vi "INIT.vi"(8 "error in (no error)":errorcluster, 11 "DAQmxTaskContainer in":refnum<class "DAQmxTaskContainer.lvclass">) -> (0 "error out":errorcluster, 3 "DAQmxTaskContainer out":refnum<class "DAQmxTaskContainer.lvclass">)   [LabVIEW 2015, in "DAQmxTaskContainer.lvclass"]
uses:
  DAQmxTaskContainer.lvclass
  dependecies/ControlsVIs/Clusters-def/SERVER-Commands.ctl
  dependecies/ControlsVIs/Clusters-def/Message types.ctl
  DAQmxTaskContainer_General/DAQmxTaksContainer_General.lvclass/DAQmxTaksContainer_General.ctl
  DAQmxTask.lvclass/DAQmxTask.ctl
  DAQmxTaskContainer_General/DAQmxTaksContainer_General.lvclass
  DAQmxTask.lvclass
  Control/Control-Server/Control-Server.lvclass
  Message/Message.lvclass
  GeneralFunctionality/GeneralFunctionality.lvclass
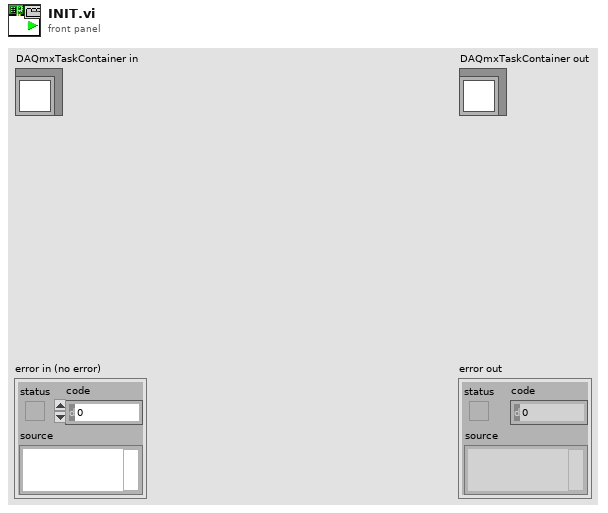
[diagram p1: front panel]
types:
  T1 = typedef "Message types.ctl" = string
  T2 = typedef "Control-Server.lvclass/SERVER-Commands.ctl" = string
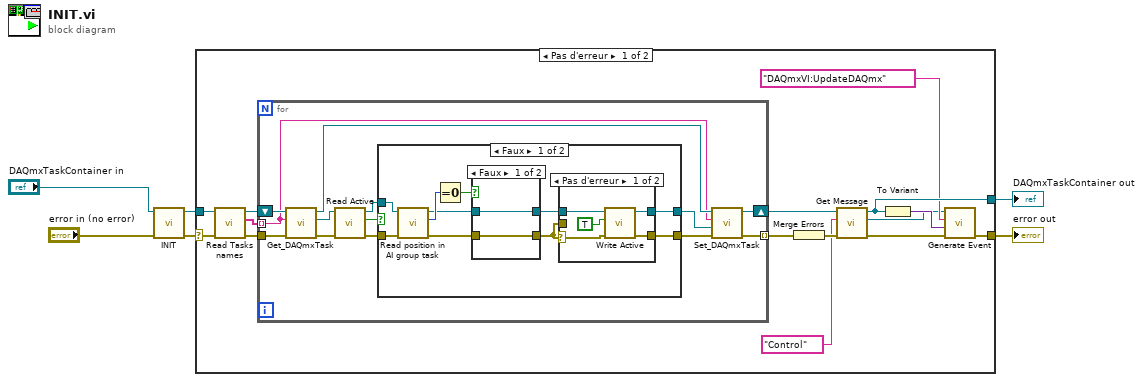
[diagram p0: block diagram]
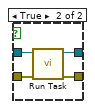
[diagram p2: hidden frame]
diagram:
  n1 = call-parent "INIT.vi"("error in (no error)"="error in (no error)", "DAQmxTaksContainer_General in"="DAQmxTaskContainer in") -> ("error out"=w4:errorcluster, "DAQmxTaksContainer_General out"=w2:refnum<class "DAQmxTaskContainer.lvclass">)  [unwired: 8 in]
  n2 = case shown="Pas d'erreur" w4 {
    selector: w4 -> [w8 w61]
    tunnel: [w17 w61] -> w3
    tunnel: [w19 w60] -> w1
    tunnel: w2 -> [w7 w60]
    frame No Error {
      n3 = call "Read Tasks names.vi"("error in (no error)"=w8, "DAQmxTaksContainer_General in"=w7) -> ("error out"=w12:errorcluster, "Tasks names"=w10:string[], "DAQmxTaksContainer_General out"=w11:refnum<class "DAQmxTaskContainer.lvclass">)  [unwired: 7 in]
      n4 = for {
        tunnel: w10 -> [w26] mode=indexing
        tunnel: w12 -> [w30]
        tunnel: [w25] -> w21 mode=indexing
        shift-right: [w23] -> w18
        shift-left: w11 -> [w31]
        n5 = call "Get_DAQmxTask.vi"("error in (no error)"=w30, "Task name"=w26, "DAQmxTaksContainer_General in"=w31) -> ("error out"=w28:errorcluster, "DAQmx Task"=w29:refnum<class "DAQmxTask.lvclass">, "DAQmxTaksContainer_General out"=w27:refnum<class "DAQmxTaskContainer.lvclass">)  [unwired: 6 in]
        n6 = call-dynamic "Read Active.vi"("error in (no error)"=w28, "DAQmxTask in"=w29) -> ("error out"=w32:errorcluster, "Active?"=w34:bool, "DAQmxTask out"=w33:refnum<class "DAQmxTask.lvclass">)  [unwired: 7 in]
        n7 = case shown="Faux" w34 {
          tunnel: w33 -> [w39 w59]
          tunnel: w32 -> [w40 w58]
          tunnel: [w44 w58] -> w24
          tunnel: [w43 w59] -> w22
          frame False {
            n8 = call "Read position in AI group task.vi"("error in (no error)"=w40, "DAQmxTask in"=w39) -> ("error out"=w37:errorcluster, "position in AI group task"=w38:i32, "DAQmxTask out"=w36:refnum<class "DAQmxTask.lvclass">)  [unwired: 7 in]
            n9 = Equal To 0?(x=w38) -> (x = 0?=w35:bool)
            n10 = case shown="Faux" w35 {
              tunnel: [w45 w50] -> w42
              tunnel: [w46 w49] -> w41
              tunnel: w37 -> [w46 w47]
              tunnel: w36 -> [w45 w48]
              frame False {
              }
              frame True {
                n11 = call "Run Task.vi"("error in (no error)"=w47, "DAQmxTask in"=w48) -> ("error out"=w49:errorcluster, "DAQmxTask out"=w50:refnum<class "DAQmxTask.lvclass">)  [unwired: 8 in]
              }
            }
            n12 = case shown="Pas d'erreur" w41 {
              selector: w41 -> [w55 _]
              tunnel: [w53 w56] -> w44
              tunnel: [w52 w57] -> w43
              tunnel: w42 -> [w51 w57]
              tunnel: w41 -> [_ w56]
              frame No Error {
                n13 = call-dynamic "Write Active.vi"("error in (no error)"=w55, "Active?"=TRUE, "DAQmxTask in"=w51) -> ("error out"=w53:errorcluster, "DAQmxTask out"=w52:refnum<class "DAQmxTask.lvclass">)  [unwired: 7 in]
              }
              frame Error {
              }
            }
          }
          frame True {
          }
        }
        n14 = call "Set_DAQmxTask.vi"("error in (no error)"=w24, "DAQmxTask"=w22, "Task name"=w26, "DAQmxTaksContainer_General in"=w27) -> ("error out"=w25:errorcluster, "DAQmxTaksContainer_General out"=w23:refnum<class "DAQmxTaskContainer.lvclass">)  [unwired: 6 in]
      }
      n15 = Merge Errors(w21) -> (w20:errorcluster)
      n16 = call "Get Message.vi"("error in (no error)"=w20, "Message type"=T1 "Control", "GeneralFunctionality en entrée"=w18) -> ("error out"=w13:errorcluster, "Message.lvclass"=w14:refnum<class "Message.lvclass">, "GeneralFunctionality en sortie"=w19:refnum<class "DAQmxTaskContainer.lvclass">)  [unwired: 6 in]
      n17 = To Variant(anything=w19) -> (Variant=w15:variant)
      n18 = call "Generate Event.vi"("error in (no error)"=w13, "Data"=w15, "Command"=T2 "DAQmxVI:UpdateDAQmx", "Message en entrée"=w14) -> ("error out"=w17:errorcluster)  [unwired: 6 in, 1 out]
    }
    frame Error {
    }
  }
  "error out" <- w3
  "DAQmxTaskContainer out" <- w1
